vi "Initiate Synchronous Generation.vi"(0 "RF Generator Handle in":refnum<k15>, 5 "Envelope Generator Handle in":refnum<k15>, 7 "Synchronization Configuration":T1={"RF Delay Range (s)"=1.9999999949504854e-06, "RF Delay (s)"=0.0} {"RF Delay (s)" format="%#_6p"; "RF Delay Range (s)" format="%#_6p"}, 11 "error in (no error)":errorcluster) -> (4 "RF Generator Handle out":refnum<k15>, 6 "Envelope Generator Handle out":refnum<k15>, 15 "error out":errorcluster)   [LabVIEW 2019, in "Envelope Tracking.lvlib"]
doc: "Synchronizes the RF and envelope signal generators, and initiates generation."
uses:
  Envelope Tracking.lvlib
  Typedefs/Synchronization Configuration.ctl
  <resource>/objmgr/sessionReference.rc
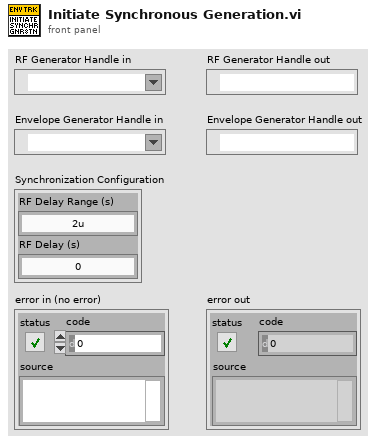
[diagram p1: front panel]
types:
  T1 = typedef "Envelope Tracking.lvlib/Synchronization Configuration.ctl" = cluster{"RF Delay Range (s)":dbl, "RF Delay (s)":dbl}
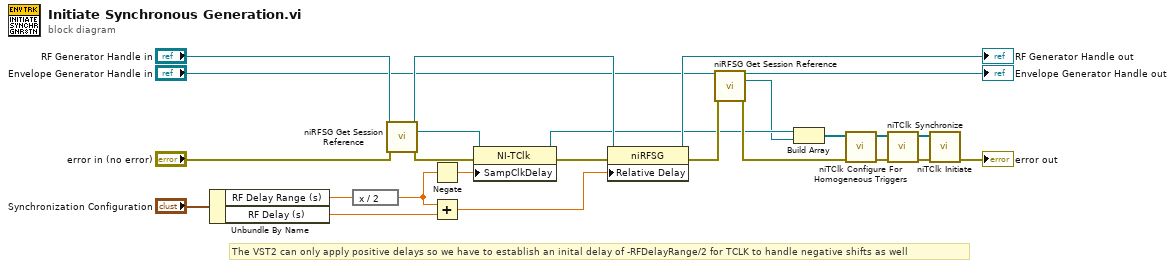
[diagram p0: block diagram]
diagram:
  # "The VST2 can only apply positive delays so we have to establish an inital delay of -RFDelayRange/2 for TCLK to handle negative shifts as well"
  n1 = Unbundle By Name("Synchronization Configuration") -> ("RF Delay Range (s)"=w2:dbl, "RF Delay (s)"=w10:dbl)
  n2 = expression code="x / 2"(w2) -> (w1:dbl)
  n3 = call <instrlib>:"niRFSG Get Session Reference.vi"("instrument handle"="RF Generator Handle in", "error in"="error in (no error)") -> ("instrument handle out"=w11:refnum<k15>, "session reference"=w6:refnum<k20>, "error out"=w22:errorcluster)  [unwired: 11 in]
  n4 = Negate(x=w1) -> (-x=w14:dbl)
  n5 = Add(x=w1, y=w10) -> (x+y=w9:dbl)
  n6 = property class="NI-TClk"(reference=w6, error in=w22, "SampClkDelay"=w14) -> (reference out=w4:refnum<k20>, error out=w21:errorcluster)
  n7 = property class="niRFSG"(reference=w11, error in=w21, "Relative Delay"=w9) -> (reference out=→"RF Generator Handle out":refnum<k15>, error out=w20:errorcluster)
  n8 = call <instrlib>:"niRFSG Get Session Reference.vi"("instrument handle"="Envelope Generator Handle in", "error in"=w20) -> ("instrument handle out"=→"Envelope Generator Handle out":refnum<k15>, "session reference"=w3:refnum<k20>, "error out"=w19:errorcluster)  [unwired: 11 in]
  n9 = Build Array(w4, w3) -> (w5:refnum<k20>[])
  n10 = call <instrlib>:"niTClk Configure For Homogeneous Triggers.vi"("error in (no error)"=w19, "sessions"=w5) -> ("error out"=w25:errorcluster, "sessions out"=w16:refnum<k20>[])  [unwired: 8 in]
  n11 = call <instrlib>:"niTClk Synchronize.vi"("error in (no error)"=w25, "sessions"=w16) -> ("error out"=w24:errorcluster, "sessions out"=w15:refnum<k20>[])  [unwired: 8 in]
  n12 = call <instrlib>:"niTClk Initiate.vi"("error in (no error)"=w24, "sessions"=w15) -> ("error out"=→"error out":errorcluster)  [unwired: 8 in, 1 out]
